vi "AMC e.bloxx Get Variable Information.vi"(8 "error in (no error)":errorcluster, 9 "Variable":i32, 10 "Module Address":i32, 11 "VISA Resource Name":refnum<visa-resource-name>) -> (0 "error out":errorcluster, 2 "Variable Information":T1={"Variable Name"="", "Variable Type"=48, "Data Format"=48, "Unit"="", "Field Length"=0, "Decimals"=0, "Host Input"=48} {"Host Input" items=["Not Possible"=48, "Possible"=49]; "Data Format" items=["No Format"=48, "Boolean"=49, "Integer"=52, "Long"=54, "Real"=56, "Set 8"=57]; "Variable Type" items=["Empty"=48, "Analog Input"=49, "Arithmetic"=50, "Digital Output"=51, "Digital Input"=52, "Setpoint"=53, "Alarm"=54, "Controller"=57]}, 3 "VISA Resource Name out":refnum<visa-resource-name>)   [LabVIEW 2013]
doc: "<B>AMC - Analytik & Messtechnik GmbH Chemnitz</B>\n\nLabVIEW Drivers for e.bloxx series from Gantner Instruments\n\nThis VI reads the variable information from the variable specified by <B>Module Address</B> and <B>Variable</B> (starts counting with 0)."
uses:
  AMC e.bloxx Variable Information.ctl
  AMC e.bloxx Variable Type.ctl
  AMC e.bloxx Data Format.ctl
  AMC e.bloxx Host Input.ctl
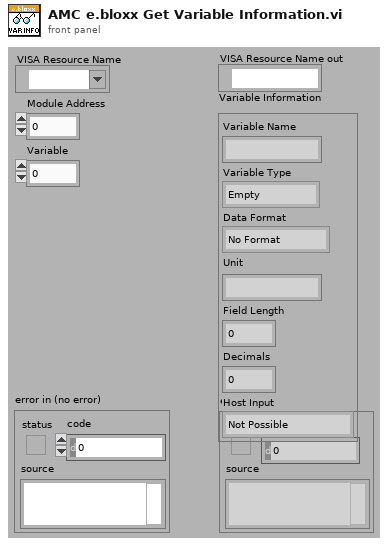
[diagram p1: front panel]
types:
  T1 = typedef "AMC e.bloxx Variable Information.ctl" = cluster{"Variable Name":string, "Variable Type":T2, "Data Format":T3, "Unit":string, "Field Length":u8, "Decimals":u8, "Host Input":T4}
  T2 = typedef "AMC e.bloxx Variable Type.ctl" = u8
  T3 = typedef "AMC e.bloxx Data Format.ctl" = u8
  T4 = typedef "AMC e.bloxx Host Input.ctl" = u8
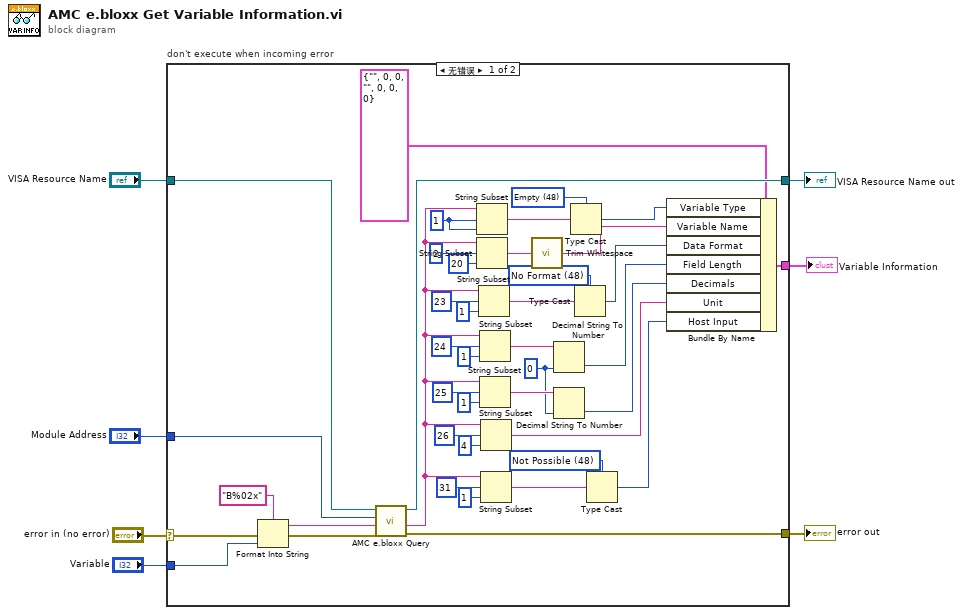
[diagram p0: block diagram]
diagram:
  n1 = case "don't execute when incoming error" shown="无错误" "error in (no error)" {
    selector: "error in (no error)" -> [w44 w51]
    tunnel: [w47 w51] -> w6
    tunnel: "VISA Resource Name" -> [w48 w50]
    tunnel: "Module Address" -> [w49 _]
    tunnel: [w46 w50] -> w3
    tunnel: "Variable" -> [w43 _]
    tunnel: [w15 _] -> w1
    frame No Error {
      w17 = T4 48 items=["Not Possible"=48, "Possible"=49] ("e.bloxx Host Input")
      w24 = u8 0
      w32 = T3 48 items=["No Format"=48, "Boolean"=49, "Integer"=52, "Long"=54, "Real"=56, "Set 8"=57] ("e.bloxx Data Format")
      w38 = T2 48 items=["Empty"=48, "Analog Input"=49, "Arithmetic"=50, "Digital Output"=51, "Digital Input"=52, "Setpoint"=53, "Alarm"=54, "Controller"=57] ("Variable Type")
      w39 = 1 ("length (rest)")
      n2 = Format Into String(format string="B%02x", error in=w44, w43) -> (resulting string=w41:string, error out=w42:errorcluster)  [unwired: 1 in]
      n3 = call "AMC e.bloxx Query.vi"("error in (no error)"=w42, "Module Command"=w41, "Module Address"=w49, "VISA Resource Name"=w48) -> ("error out"=w47:errorcluster, "Module Response"=w21:string, "VISA Resource Name out"=w46:refnum<visa-resource-name>)  [unwired: 5 in]
      n4 = String Subset(string=w21, offset (0)=w39, length (rest)=w39) -> (substring=w40:string)
      n5 = String Subset(string=w21, offset (0)=2, length (rest)=20 ("length (rest)")) -> (substring=w35:string)
      n6 = String Subset(string=w21, offset (0)=23, length (rest)=1 ("length (rest)")) -> (substring=w31:string)
      n7 = String Subset(string=w21, offset (0)=24, length (rest)=1 ("length (rest)")) -> (substring=w26:string)
      n8 = String Subset(string=w21, offset (0)=25, length (rest)=1 ("length (rest)")) -> (substring=w25:string)
      n9 = String Subset(string=w21, offset (0)=26, length (rest)=4 ("length (rest)")) -> (substring=w9:string)
      n10 = String Subset(string=w21, offset (0)=31, length (rest)=1 ("length (rest)")) -> (substring=w18:string)
      n11 = call <vilib>:"Trim Whitespace.vi"("string"=w35) -> ("trimmed string"=w13:string)  [unwired: 1 in]
      n12 = Decimal String To Number(string=w26, default (0L)=w24) -> (number=w11:u8)  [unwired: 1 in, 1 out]
      n13 = Decimal String To Number(string=w25, default (0L)=w24) -> (number=w10:u8)  [unwired: 1 in, 1 out]
      n14 = Type Cast(type=w38, x=w40) -> (*(type *) &x=w14:T2)
      n15 = Type Cast(type=w32, x=w31) -> (*(type *) &x=w12:T3)
      n16 = Type Cast(type=w17, x=w18) -> (*(type *) &x=w8:T4)
      n17 = Bundle By Name(cluster=T1 {"Variable Name"="", "Variable Type"=0, "Data Format"=0, "Unit"="", "Field Length"=0, "Decimals"=0, "Host Input"=0} ("Variable Information"), "Variable Type"=w14, "Variable Name"=w13, "Data Format"=w12, "Field Length"=w11, "Decimals"=w10, "Unit"=w9, "Host Input"=w8) -> (w15:T1)
    }
    frame Error {
    }
  }
  "error out" <- w6
  "VISA Resource Name out" <- w3
  "Variable Information" <- w1
